vi "test_VI Set_Get Protocol VISA.vi"(8 "error in (no error)":errorcluster, 11 "TestCase in":refnum<class "Instrument Addon Scripting API Custom Device Unit Tests.lvclass">) -> (0 "error out":errorcluster, 3 "TestCase out":refnum<class "Instrument Addon Scripting API Custom Device Unit Tests.lvclass">)   [LabVIEW 2018, in "Instrument Addon Scripting API Custom Device Unit Tests.lvclass"]
uses:
  Instrument Addon Scripting API Custom Device Unit Tests.lvclass
  Addon/Support Libraries/Protocols.lvlibp/VISA/VISA.lvclass
  C:/Users/nitest/Git/NI VS Instrument Addon Fork/Source/Addon/Support Libraries/Protocols.lvlibp/Protocol Parent/Protocol Parent.lvclass
  NationalInstruments.VeriStand.SystemDefinitionAPI
  Addon/Support Libraries/Protocols.lvlibp/VISA/Data Access/Write Append Write Termination Character.vi
  Addon/Support Libraries/Protocols.lvlibp/VISA/Data Access/Write Enable Termination Character.vi
  Addon/Support Libraries/Protocols.lvlibp/VISA/Data Access/Write Termination Character.vi
  Addon/Support Libraries/Protocols.lvlibp/VISA/Data Access/Write Timeout.vi
  Addon/Support Libraries/Protocols.lvlibp/VISA/Data Access/Write VISA Resource.vi
  Instrument Addon Scripting API Test Assets/Instrument Addon Scripting API Test Assets.lvclass
  <vilib>/addons/_JKI Toolkits/VI Tester/TestCase.llb/TestCase.lvclass
  APIs/Scripting API/Instrument Addon Scripting API.lvlib
  C:/Program Files (x86)/National Instruments/LabVIEW 2018/vi.lib/addons/_JKI Toolkits/VI Tester/TestCase.llb/TestCase.lvclass
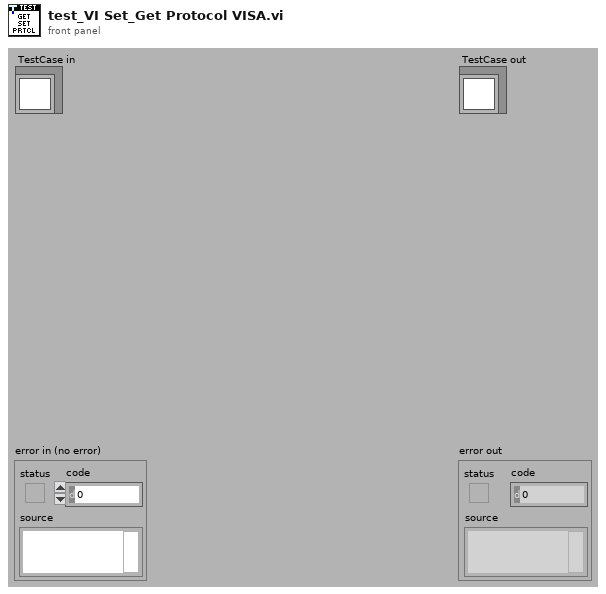
[diagram p1: front panel]
types:
  T1 = typedef "Custom Device API.lvlib/Custom Device Item Ref.ctl" = u64
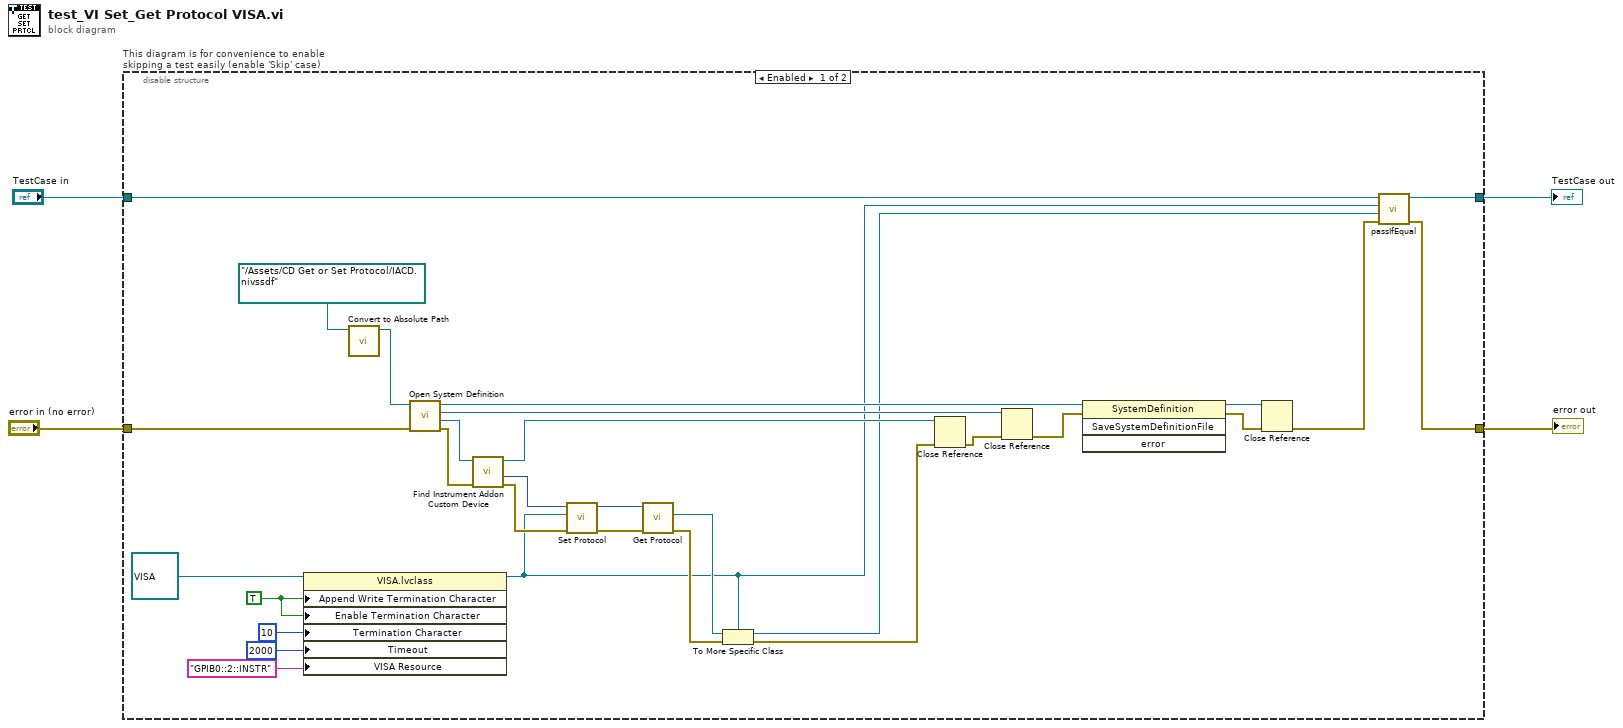
[diagram p0: block diagram]
diagram:
  n1 = disable-structure "This diagram is for convenience to enable skipping a test easily (enable 'Skip' case)" shown="Enabled" {
    disable-tunnel: "TestCase in" -> [w10 w38]
    disable-tunnel: [w9 w36] -> w1
    disable-tunnel: [w5 w37] -> w3
    disable-tunnel: "error in (no error)" -> [w34 w35]
    frame Enabled {
      w17 = TRUE
      n2 = property class="VISA.lvclass"(reference=refnum<class "VISA.lvclass"> refnum ("Protocols.lvlibp:VISA.lvclass"), "Append Write Termination Character"=w17, "Enable Termination Character"=w17, "Termination Character"=u8 10, "Timeout"=u32 2000, "VISA Resource"="GPIB0::2::INSTR") -> (reference out=w7:refnum<class "VISA.lvclass">)  [unwired: 1 in, 1 out]
      n3 = call "Convert to Absolute Path.vi"("System Definition File"=path "../Assets/CD Get or Set Protocol/IACD.nivssdf" ("SDF file")) -> ("Absolute Path"=w32:path)  [unwired: 10 in]
      n4 = call "Open System Definition.vi"("error in (no error)"=w34, "System Definition File"=w32) -> ("error out"=w29:errorcluster, "Target Refnum"=w28:refnum<k24>, "Root Refnum"=w31:refnum<k24>, "System Definition Refnum"=w22:refnum<k24>)  [unwired: 6 in]
      n5 = call "Find Instrument Addon Custom Device.vi"("error in"=w29, "target in"=w28) -> ("error out"=w27:errorcluster, "NodeID"=w26:u64, "target out"=w25:refnum<k24>)  [unwired: 7 in]
      n6 = call "Set Protocol.vi"("Error In"=w27, "Protocol in"=w7, "Instrument Addon Refnum In"=w26) -> ("Error Out"=w23:errorcluster, "Instrument Addon Refnum Out"=w24:T1)  [unwired: 7 in]
      n7 = call "Get Protocol.vi"("Error In"=w23, "Instrument Addon Refnum In"=w24) -> ("Error Out"=w13:errorcluster, "Protocol"=w14:refnum<class "Protocol Parent.lvclass">)  [unwired: 7 in, 1 out]
      n8 = To More Specific Class(target class=w7, reference=w14, error in=w13) -> (specific class reference=w8:refnum<class "VISA.lvclass">, error out=w11:errorcluster)
      n9 = Close Reference(reference=w25, error in (no error)=w11) -> (error out=w30:errorcluster)
      n10 = Close Reference(reference=w31, error in (no error)=w30) -> (error out=w21:errorcluster)
      n11 = invoke class="SystemDefinition" method="SaveSystemDefinitionFile"(reference=w22, error in=w21) -> (reference out=w20:refnum<k24>, error out=w19:errorcluster)  [unwired: 2 in, 2 out]
      n12 = Close Reference(reference=w20, error in (no error)=w19) -> (error out=w6:errorcluster)
      n13 = call-dynamic "passIfEqual.vi"("error in (no error)"=w6, "y"=w8, "x"=w7, "TestCase in"=w10) -> ("error out"=w5:errorcluster, "TestCase out"=w9:refnum<class "Instrument Addon Scripting API Custom Device Unit Tests.lvclass">)  [unwired: 6 in]
    }
    frame Disabled {
      # "skip test result while test is under development"
      n14 = call <vilib>:"skip.vi"("error in (no error)"=w35, "TestCase in"=w38) -> ("error out"=w37:errorcluster, "TestCase out"=w36:refnum<class "Instrument Addon Scripting API Custom Device Unit Tests.lvclass">)  [unwired: 8 in]
    }
  }
  "error out" <- w3
  "TestCase out" <- w1
